vi "DSP_GetPostTrigCfg.vi"() -> ()   [LabVIEW 2009]
panel:
  out "value":u32
  out "error out":errorcluster
  in  "error in (no error)":errorcluster
  out "Board Handle Out":u64
  in  "Board Handle":u64
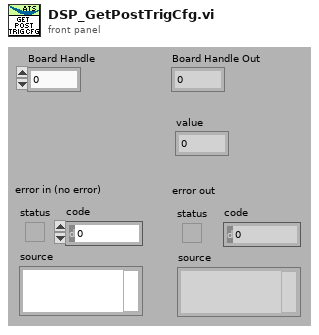
[diagram p1: front panel]
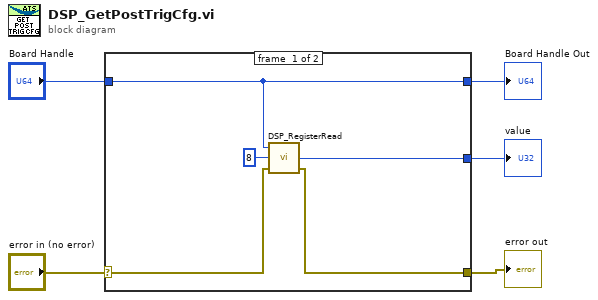
[diagram p0: block diagram]
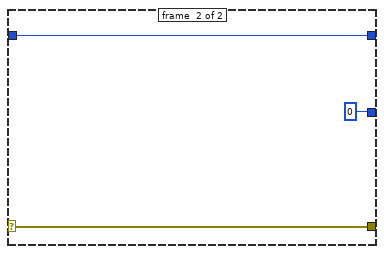
[diagram p2: hidden frame]
diagram:
  n1 = case shown="No Error" "error in (no error)" {
    selector: "error in (no error)" -> [w9 w13]
    tunnel: [w8 w13] -> w4
    tunnel: [w10 w12] -> w3
    tunnel: "Board Handle" -> [w10 w12]
    tunnel: [w6 u32 0] -> w1
    frame #0 {
      n2 = call "DSP_RegisterRead.vi"("error in (no error)"=w9, "Offset"=u32 8, "Board Handle"=w10) -> ("error out"=w8:errorcluster, "Value"=w6:u32)  [unwired: 1 out]
    }
    frame #1 {
    }
  }
  "Board Handle Out" <- w3
  "error out" <- w4
  "value" <- w1
